vi "Log.vi"(0 "Logger Mananger in":refnum<class "Logger Mananger.lvclass">, 5 "Log Level":T1, 7 "Caller":string, 9 "Msg":string, 11 "error in (no error)":errorcluster) -> (4 "Logger Mananger out":refnum<class "Logger Mananger.lvclass">, 15 "error out":errorcluster)   [LabVIEW 2020, in "Logging.lvlib" / "Logger Mananger.lvclass"]
uses:
  Logger Mananger.lvclass
  Define/Log Level.ctl
  Logger Mananger.lvclass/Logger Mananger.ctl
  Generic Logger Messages/Logging Msg/Logging Msg.lvclass/Logging Msg.ctl
  <vilib>/ActorFramework/Message Enqueuer/Message Enqueuer.lvclass/Message Enqueuer.ctl
  <vilib>/ActorFramework/Message Enqueuer/Enqueue.vi
  Generic Logger Messages/Logging Msg/Logging Msg.lvclass
  C:/Program Files (x86)/National Instruments/LabVIEW 2020/vi.lib/ActorFramework/Message/Message.lvclass
  <vilib>/ActorFramework/Message Priority Queue/Priority Enqueue.vi
  Logging.lvlib
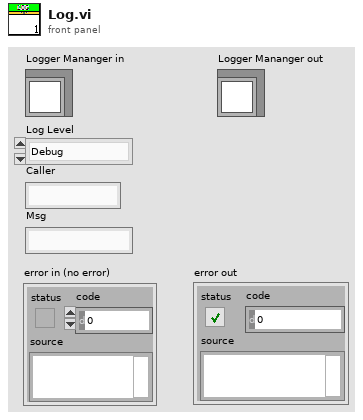
[diagram p1: front panel]
types:
  T1 = typedef "Logging.lvlib/Log Level.ctl" = enum16{"Debug", "Info", "Warn", "Error"}
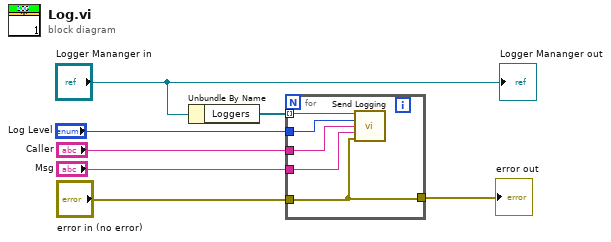
[diagram p0: block diagram]
diagram:
  n1 = Unbundle By Name("Logger Mananger in") -> ("Loggers"=w6:refnum<class "Message Enqueuer.lvclass">[])
  n2 = for {
    tunnel: w6 -> [w12] mode=indexing
    tunnel: "Log Level" -> [w11]
    tunnel: "Msg" -> [w10]
    tunnel: "Caller" -> [w9]
    tunnel: "error in (no error)" -> [w8]
    tunnel: [w8] -> w1
    n3 = call "Send Logging.vi"("Message Enqueuer"=w12, "Log Level"=w11, "Caller"=w9, "Content"=w10, "error in (no error)"=w8) -> ()  [unwired: 9 in, 2 out]
  }
  "error out" <- w1
  "Logger Mananger out" <- "Logger Mananger in"
